vi "IMAQ Image to 2d u32.vi"(0 "Image":T1, 5 "error in (no error)":errorcluster) -> (14 "Image Pixels (U32)":u32[][](array[numeric]), 19 "error out":errorcluster)   [LabVIEW 2015]
uses:
  <vilib>/vision/Image Controls.llb/IMAQ Image.ctl
  nivissvc.dll
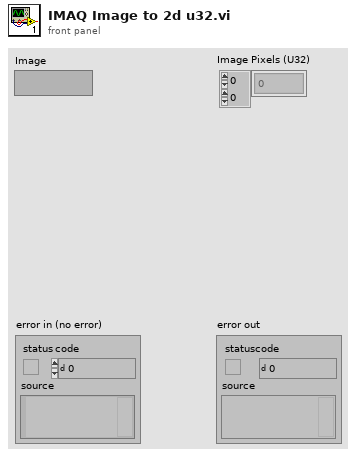
[diagram p1: front panel]
types:
  T1 = typedef "IMAQ Image.ctl" = refnum<image>
  T2 = cluster{"Plane 3 (Blue)":u8, "Plane 2 (Green)":u8, "Plane 1 (Red)":u8, "Plane 4 (alpha)":u8}[][]
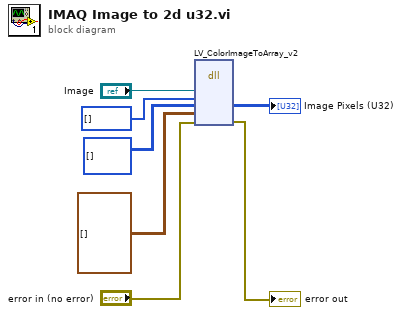
[diagram p0: block diagram]
diagram:
  n1 = dll-call lib="nivissvc.*" fn="LV_ColorImageToArray_v2"("image"="Image", "region"=i32[] [] ("Optional Rectangle"), "imagePixels32"=u32[][] [] ("Image Pixels (U32)"), "imagePixels64"=T2 [] ("Image Pixels (U64)"), "error"="error in (no error)") -> ("imagePixels32"=→"Image Pixels (U32)":u32[][], "error"=→"error out":errorcluster)  [unwired: 5 in, 4 out]
